vi "UART_U8_Open.vi"(6 "stop bits (10: 1 bit)":u16(ring)=10 items=["1.0"=10, "1.5"=15, "2.0"=20], 8 "error in":errorcluster, 9 "parity (0:none)":enum16{"None", "Odd", "Even", "Mark", "Space"}(ring), 10 "baud rate (115200)":u32=19200, 11 "VISA resource name":refnum<visa-resource-name>="COM1") -> (0 "error out":errorcluster, 3 "VISA resource name out":refnum<visa-resource-name>="COM1")   [LabVIEW 2015, in "UARTCOM.lvlib"]
uses:
  UARTCOM.lvlib
  <vilib>/Instr/_visa.llb/VISA Configure Serial Port (Instr).vi
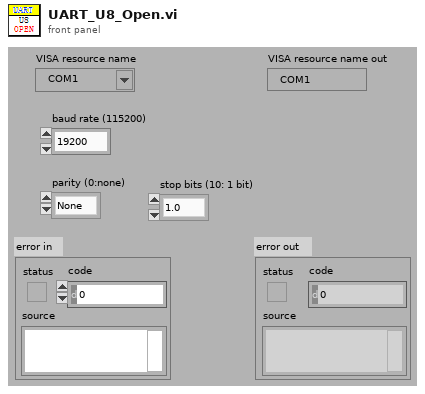
[diagram p1: front panel]
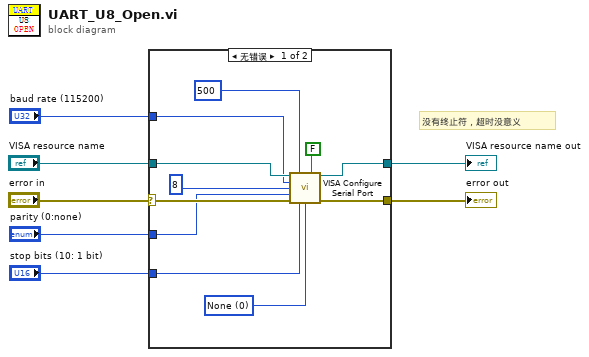
[diagram p0: block diagram]
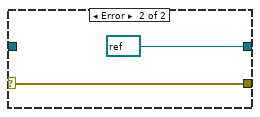
[diagram p2: hidden frame]
diagram:
  # "没有终止符，超时没意义"
  n1 = case shown="无错误" "error in" {
    selector: "error in" -> [w16 w20]
    tunnel: [w18 w20] -> w6
    tunnel: [w17 refnum<visa-resource-name> refnum ("VISA resource name out")] -> w4
    tunnel: "VISA resource name" -> [w15 _]
    tunnel: "baud rate (115200)" -> [w12 _]
    tunnel: "parity (0:none)" -> [w11 _]
    tunnel: "stop bits (10: 1 bit)" -> [w8 _]
    frame No Error {
      w13 = u16 0 items=["None", "XON/XOFF", "RTS/CTS", "XON/XOFF & RTS/CTS", "DTR/DSR", "XON/XOFF & DTR/DSR"] ("flow control (0:none)")
      n2 = call-poly "VISA Configure Serial Port"("VISA resource name"=w15, "timeout (10sec)"=u32 500, "Enable Termination\nChar (T)"=FALSE ("Enable Termination\nChar (T)"), "baud rate (9600)"=w12, "data bits (8)"=u16 8, "parity (0:none)"=w11, "error in (no error)"=w16, "stop bits (10: 1 bit)"=w8, "flow control (0:none)"=w13) -> ("VISA resource name out"=w17:refnum<visa-resource-name>, "error out"=w18:errorcluster)  [unwired: 5 in]
    }
    frame Error {
    }
  }
  "error out" <- w6
  "VISA resource name out" <- w4
